vi "2D Inverse DCT.vi"(11 "DCT {X}":dbl[][](array[numeric])) -> (0 "error":i32, 3 "X":dbl[][](array[numeric]))   [LabVIEW 2010, in "NI_AALPro.lvlib"]
doc: "Computes the inverse Discrete Cosine Transform (DCT) of the input sequence <B>DCT {X}</B>. Wire data to the <B>DCT {X}</B> input to determine the polymorphic instance to use or manually select the instance."
uses:
  NI_AALPro.lvlib
  lvanlys.dll
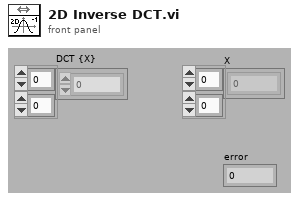
[diagram p1: front panel]
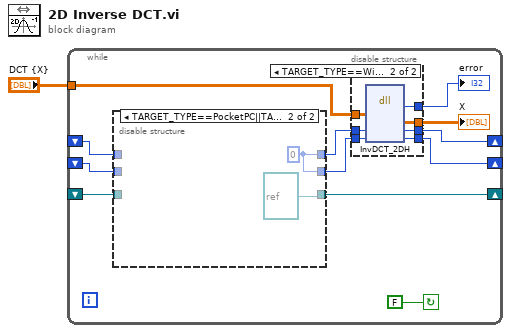
[diagram p0: block diagram]
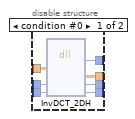
[diagram p2: hidden frame]
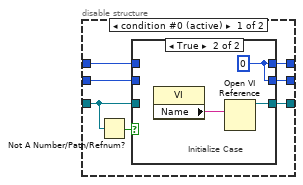
[diagram p3: hidden frame]
diagram:
  n1 = while {
    shift-left: _ -> [w11]
    shift-right: [w6] -> _
    tunnel: "DCT {X}" -> [w12]
    shift-right: [w10] -> _
    shift-left: _ -> [w9]
    shift-right: [w4] -> _
    shift-left: _ -> [w3]
    stop <- FALSE continue-if-true
    n2 = disable-structure shown="TARGET_TYPE==PocketPC||TARGET_TYPE==PalmOS||TARGET_TYPE==FPGA||TARGET_TYPE==Embedded" {
      disable-tunnel: w9 -> [w32 _]
      disable-tunnel: [w33 refnum<vi> refnum ("VI Refnum")] -> w10
      disable-tunnel: w11 -> [w31 _]
      disable-tunnel: [w30 w42] -> w7
      disable-tunnel: w3 -> [w29 _]
      disable-tunnel: [w28 w42] -> w2
      frame condition #0 (active) {
        n3 = Not A Number/Path/Refnum?(number/path/refnum=w32) -> (NaN/Path/Refnum?=w34:bool)
        n4 = case shown="True" w34 {
          tunnel: [w37 w40] -> w33
          tunnel: w32 -> [w37 _]
          tunnel: w31 -> [w36 _]
          tunnel: [w36 w39] -> w30
          tunnel: w29 -> [w35 _]
          tunnel: [w35 w39] -> w28
          frame False {
          }
          frame True {
            w39 = 0 ("error")
            # "Initialize Case"
            n5 = property class="VI"() -> ("Name"=w38:string)  [unwired: 2 in, 2 out]
            n6 = Open VI Reference(vi path=w38) -> (vi reference=w40:refnum<vi>)  [unwired: 5 in, 1 out]
          }
        }
      }
      frame condition #1 {
        w42 = 0 ("t")
      }
    }
    n7 = disable-structure shown="TARGET_TYPE==Windows||TARGET_TYPE==Mac||TARGET_TYPE==Unix" {
      disable-tunnel: w12 -> [w20 w27]
      disable-tunnel: [w19 w26] -> w8
      disable-tunnel: w7 -> [w18 w25]
      disable-tunnel: [w17 w24] -> w6
      disable-tunnel: [w16 w23] -> w5
      disable-tunnel: [w15 w22] -> w4
      disable-tunnel: w2 -> [w14 w21]
      frame condition #0 {
        n8 = dll-call lib="C:/Program Files/National Instruments/LabVIEW 2010/resource/lvanlys.*" fn="InvDCT_2DH"("xH"=w20, "tbl1"=w18, "tbl2"=w14) -> (w19:i32, "yH"=w16:dbl[][], "tbl1"=w17:i32, "tbl2"=w15:i32)  [unwired: 5 in, 2 out]
      }
      frame condition #1 (active) {
        n9 = dll-call lib="C:/Program Files/National Instruments/LabVIEW 2010/resource/lvanlys.dll" fn="InvDCT_2DH"("xH"=w27, "tbl1"=w25, "tbl2"=w21) -> ("return type"=w26:i32, "yH"=w23:dbl[][], "tbl1"=w24:i64, "tbl2"=w22:i64)  [unwired: 5 in, 2 out]
      }
    }
    "error" <- w8
    "X" <- w5
  }
